vi "NanotecSMCPDDriver.set limit switch polarity.vi"(0 "VISA resource name":refnum<visa-resource-name>, 1 "contollerID":i32=-1, 3 "normallyClosed":bool, 5 "error in (no error)":errorcluster) -> (14 "VISA resource name out":refnum<visa-resource-name>, 15 "contollerID out":i32=-1, 19 "error out":errorcluster)   [LabVIEW 2014, in "NanotecSMCPDDriver.lvlib"]
doc: "Sets the polarity of the limit switch (opening or closing)."
uses:
  NanotecSMCPDDriver.lvlib
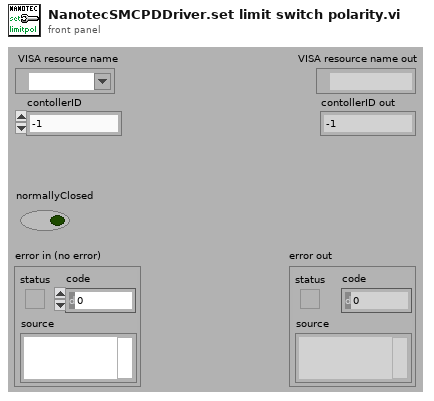
[diagram p1: front panel]
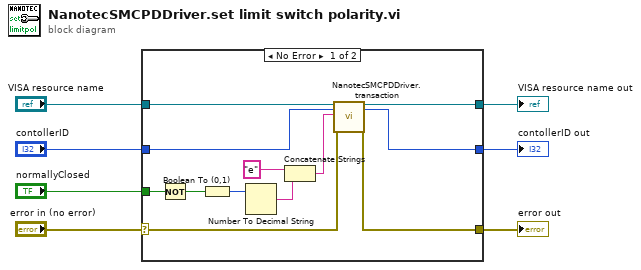
[diagram p0: block diagram]
diagram:
  n1 = case shown="No Error" "error in (no error)" {
    selector: "error in (no error)" -> [w14 w20]
    tunnel: [w16 w22] -> w7
    tunnel: [w15 w20] -> w6
    tunnel: "VISA resource name" -> [w19 w22]
    tunnel: "contollerID" -> [w18 w21]
    tunnel: [w17 w21] -> w3
    tunnel: "normallyClosed" -> [w10 _]
    frame No Error {
      n2 = Not(x=w10) -> (.not. x?=w8:bool)
      n3 = Boolean To (0,1)(Boolean=w8) -> (0, 1=w9:i16)
      n4 = Number To Decimal String(number=w9) -> (decimal integer string=w13:string)  [unwired: 1 in]
      n5 = Concatenate Strings("e" ("commandString"), w13) -> (w11:string)
      n6 = call "NanotecSMCPDDriver.transaction.vi"("VISAresource"=w19, "contollerID"=w18, "commandString"=w11, "error in (no error)"=w14) -> ("VISAresource out"=w16:refnum<visa-resource-name>, "contollerID out"=w17:i32, "error out"=w15:errorcluster)  [unwired: 10 in, 3 out]
    }
    frame Error {
    }
  }
  "VISA resource name out" <- w7
  "error out" <- w6
  "contollerID out" <- w3
